vi "Register Core gRPC Server.vi"(8 "error in (no error)":errorcluster, 10 "gRPC ID":T1, 11 "CIFTemplateNode in":refnum<class "CIFTemplateNode.lvclass">) -> (0 "error out":errorcluster, 2 "gRPC ID Out":T1, 3 "CIFTemplateNode out":refnum<class "CIFTemplateNode.lvclass">)   [LabVIEW 2021, in "CIFTemplateNode.lvclass"]
uses:
  CIFTemplateNode.lvclass
  CIFTemplateNode.lvclass/CIFTemplateNode.ctl
  CIFTemplateGrpc/CIF_Plugin_Core_server/CIF_Plugin_Core_server.lvlib
  CIFTemplateGrpc/CIF_Plugin_Core_server/RPC Service/PluginCore/PluginCore.lvclass
  <vilib>/gRPC/LabVIEW gRPC Library/Shared/grpcId.ctl
  <vilib>/gRPC/LabVIEW gRPC Library/grpc-lvsupport-release.lvlib
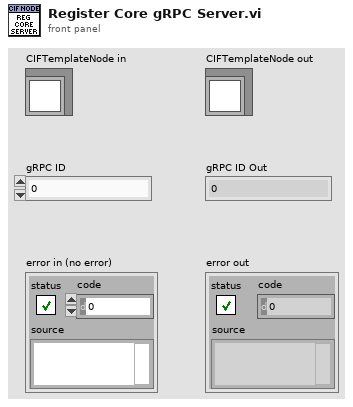
[diagram p1: front panel]
types:
  T1 = typedef "grpc-lvsupport-release.lvlib/grpcId.ctl" = u64
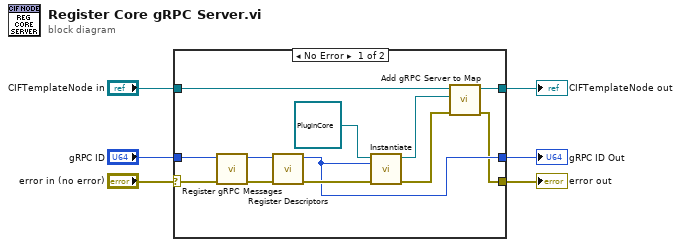
[diagram p0: block diagram]
diagram:
  n1 = case shown="No Error" "error in (no error)" {
    selector: "error in (no error)" -> [w16 w21]
    tunnel: [w7 w21] -> w5
    tunnel: [w12 w20] -> w3
    tunnel: "CIFTemplateNode in" -> [w13 w20]
    tunnel: "gRPC ID" -> [w15 w19]
    tunnel: [w8 w19] -> w1
    frame No Error {
      n2 = call "Register gRPC Messages.vi"("error in (no error)"=w16, "gRPC ID"=w15) -> ("error out"=w17:errorcluster, "gRPC ID Out"=w18:T1)  [unwired: 8 in]
      n3 = call "Register Descriptors.vi"("error in (no error)"=w17, "gRPC ID"=w18) -> ("error out"=w14:errorcluster, "gRPC ID Out"=w8:T1)  [unwired: 8 in]
      n4 = call-dynamic "Instantiate.vi"("error in"=w14, "gRPCid"=w8, "iService"=refnum<class "PluginCore.lvclass"> refnum ("CIF_Plugin_Core_server.lvlib:PluginCore.lvclass")) -> ("error out"=w10:errorcluster, "iService"=w9:refnum<class "PluginCore.lvclass">)  [unwired: 7 in]
      n5 = call "Add gRPC Server to Map.vi"("error in (no error)"=w10, "gRPC Server Class"=w9, "CIFTemplateNode in"=w13) -> ("error out"=w7:errorcluster, "CIFTemplateNode out"=w12:refnum<class "CIFTemplateNode.lvclass">)  [unwired: 7 in]
    }
    frame Error {
    }
  }
  "error out" <- w5
  "CIFTemplateNode out" <- w3
  "gRPC ID Out" <- w1
